vi "Autofocus.vi"(0 "Pos X":i32, 5 "Pos Y":i32, 9 "Cen X":i32, 11 "Cen Y":i32, 12 "a0":dbl, 13 "a1":dbl, 14 "a2":dbl) -> (8 "Foyer":i32)   [LabVIEW 2010]
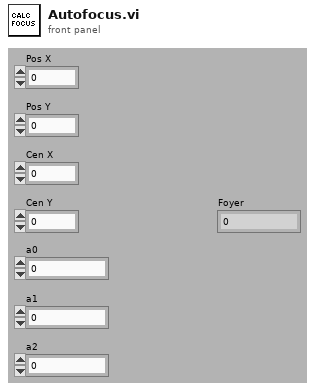
[diagram p1: front panel]
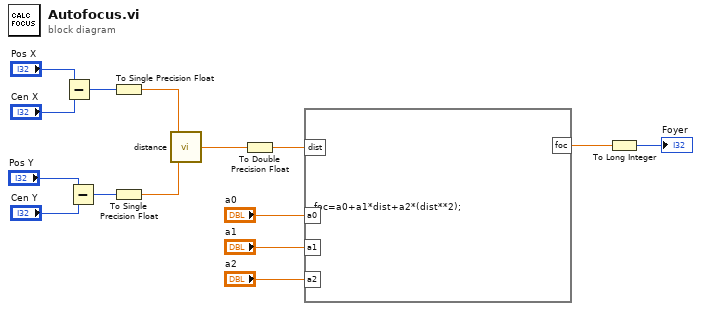
[diagram p0: block diagram]
diagram:
  n1 = Subtract(x="Pos X", y="Cen X") -> (x-y=w11:i32)
  n2 = Subtract(x="Pos Y", y="Cen Y") -> (x-y=w10:i32)
  n3 = To Single Precision Float(number=w11) -> (single precision float=w9:sgl)
  n4 = To Single Precision Float(number=w10) -> (single precision float=w8:sgl)
  n5 = call "distance.vi"("D2"=w8, "D1"=w9) -> ("DT"=w7:dbl)
  n6 = To Double Precision Float(number=w7) -> (double precision float=w6:dbl)
  n7 = formula code="foc=a0+a1*dist+a2*(dist**2);"("dist"=w6, "a0"="a0", "a1"="a1", "a2"="a2") -> ("foc"=w2:dbl)
  n8 = To Long Integer(number=w2) -> (32bit integer=→"Foyer":i32)
